vi "DSF.Memory.Buffer.Config.New.vi"(8 "error in (no error)":errorcluster, 10 "channel count":u64 format="%d channels", 11 "Buffer Config in":refnum<class "DSF.Memory.Buffer.Config.lvclass">) -> (0 "error out":errorcluster, 3 "Buffer Config out":refnum<class "DSF.Memory.Buffer.Config.lvclass">)   [LabVIEW 2016, in "DSF.Engine.lvlib" / "DSF.Memory.Buffer.Config.lvclass"]
uses:
  DSF.Memory.Buffer.Config.lvclass
  DSF.Memory.Buffer.Config.lvclass/DSF.Memory.Buffer.Config.ctl
  Memory.Pointer/DSF.Memory.Pointer.U64.lvclass
  C:/Git/SourceTree/DSF/Source/Submodules/Memory Manager/Source/Classes/Pointer.Internal/Memory.Pointer.Internal.lvclass
  Submodules/Memory Manager/Source/Classes/Pointer.Internal/Methods/Memory.Pointer.Internal.Allocate.vi
  Memory.Pointer/DSF.Engine.Memory.Pointer.DataType.lvclass
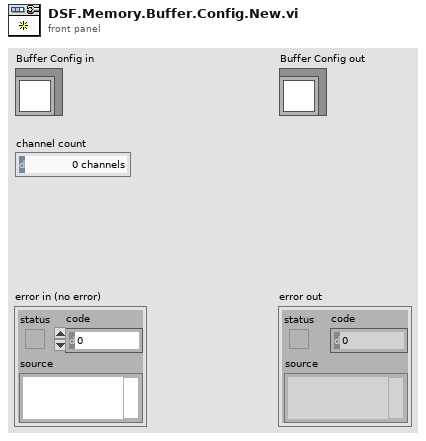
[diagram p1: front panel]
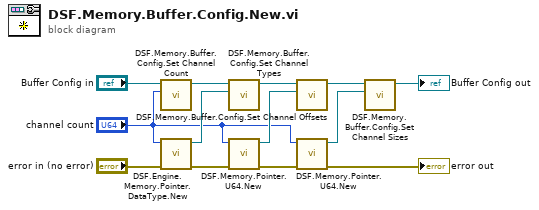
[diagram p0: block diagram]
diagram:
  n1 = call "DSF.Memory.Buffer.Config.Set Channel Count.vi"("channel count"="channel count", "Buffer Config in"="Buffer Config in") -> ("Buffer Config out"=w9:refnum<class "DSF.Memory.Buffer.Config.lvclass">)  [unwired: 8 in, 1 out]
  n2 = call "DSF.Engine.Memory.Pointer.DataType.New.vi"("error in (no error)"="error in (no error)", "count (1)"="channel count") -> ("error out"=w12:errorcluster, "Data Type pointer"=w5:refnum<class "DSF.Engine.Memory.Pointer.DataType.lvclass">)  [unwired: 8 in]
  n3 = call "DSF.Memory.Buffer.Config.Set Channel Types.vi"("channel types ptr"=w5, "Buffer Config in"=w9) -> ("Buffer Config out"=w8:refnum<class "DSF.Memory.Buffer.Config.lvclass">)  [unwired: 8 in, 1 out]
  n4 = call "DSF.Memory.Pointer.U64.New.vi"("error in (no error)"=w12, "count (1)"="channel count") -> ("error out"=w11:errorcluster, "pointer"=w4:refnum<class "DSF.Memory.Pointer.U64.lvclass">)  [unwired: 8 in]
  n5 = call "DSF.Memory.Buffer.Config.Set Channel Offsets.vi"("channel offsets ptr"=w4, "Buffer Config in"=w8) -> ("Buffer Config out"=w7:refnum<class "DSF.Memory.Buffer.Config.lvclass">)  [unwired: 8 in, 1 out]
  n6 = call "DSF.Memory.Pointer.U64.New.vi"("error in (no error)"=w11, "count (1)"="channel count") -> ("error out"=→"error out":errorcluster, "pointer"=w3:refnum<class "DSF.Memory.Pointer.U64.lvclass">)  [unwired: 8 in]
  n7 = call "DSF.Memory.Buffer.Config.Set Channel Sizes.vi"("channel sizes ptr"=w3, "Buffer Config in"=w7) -> ("Buffer Config out"=→"Buffer Config out":refnum<class "DSF.Memory.Buffer.Config.lvclass">)  [unwired: 8 in, 1 out]
